vi "PID_Separate.vi"() -> ()   [LabVIEW 2018]
uses:
  <vilib>/addons/control/pid/NI_PID_pid.lvlib
  <vilib>/addons/control/pid/pid.llb/PID (DBL).vi
panel:
  in  "Reset Encoders":bool
  in  "Vasen":dbl format="%.2f"
  in  "Oikea":dbl format="%.2f"
  in  "Taka":dbl format="%.2f"
  in  "Etu":dbl format="%.2f"
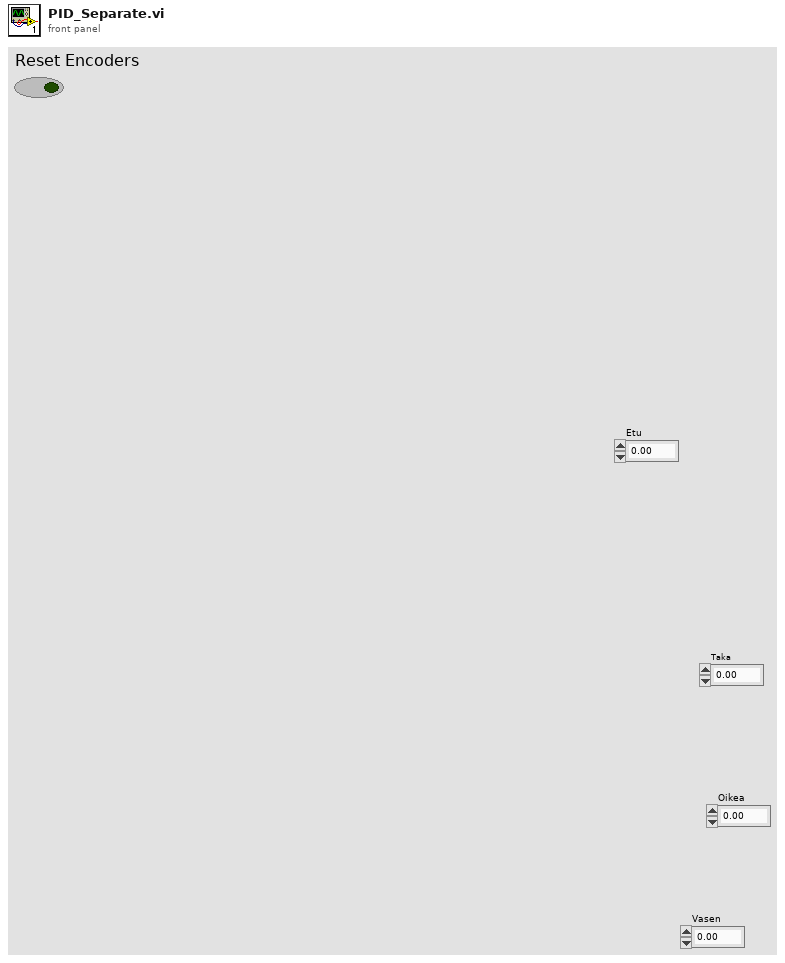
[diagram p1: front panel]
types:
  T1 = cluster{bool, "Tick Count(uSec)":u32, "Counter Value":i32[], "x-y":i32[]}
  T2 = cluster{"Position":i32[], "Velocity RPM":dbl[], "Velocity RPS":dbl[], "Radians/s":dbl[]}
  T3 = cluster{"proportional gain (Kc)":dbl, "integral time (Ti, min)":dbl, "derivative time (Td, min)":dbl}
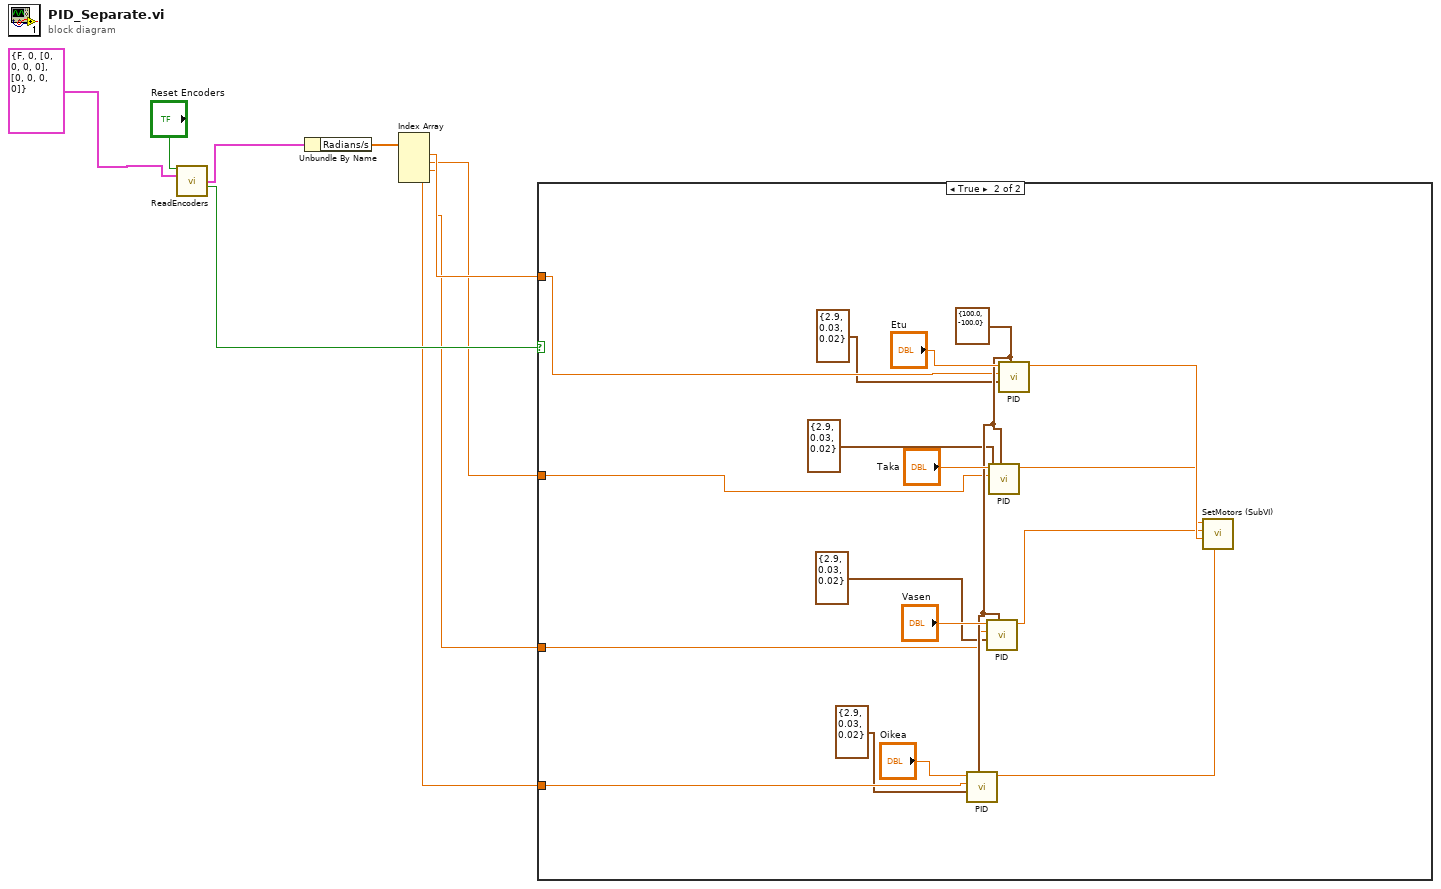
[diagram p0: block diagram]
diagram:
  n1 = call "ReadEncoders.vi"("Reset Encoders"="Reset Encoders", "Cluster in"=T1 {FALSE, "Tick Count(uSec)"=0, "Counter Value"=[0, 0, 0, 0], "x-y"=[0, 0, 0, 0]}) -> ("output cluster"=w6:T2, "Updated"=w8:bool)  [unwired: 9 in, 3 out]
  n2 = Unbundle By Name(w6) -> ("Radians/s"=w5:dbl[])
  n3 = Index Array(array=w5) -> (element #1=w4:dbl, element #2=w3:dbl, element #3=w2:dbl, element #4=w1:dbl)  [unwired: 4 in]
  n4 = case shown="True" w8 {
    tunnel: w4 -> [_ w17]
    tunnel: w3 -> [_ w16]
    tunnel: w2 -> [_ w15]
    tunnel: w1 -> [_ w14]
    frame False {
    }
    frame True {
      w18 = cluster{"output high":dbl, "output low":dbl} {"output high"=100.0, "output low"=-100.0} ("output range")
      n5 = call-poly <vilib>:"PID.vi"("output range"=w18, "PID gains"=T3 {"proportional gain (Kc)"=2.9, "integral time (Ti, min)"=0.03, "derivative time (Td, min)"=0.02}, "process variable"=w14, "setpoint"="Oikea") -> ("output"=w19:dbl)  [unwired: 6 in, 1 out]
      n6 = call-poly <vilib>:"PID.vi"("output range"=w18, "PID gains"=T3 {"proportional gain (Kc)"=2.9, "integral time (Ti, min)"=0.03, "derivative time (Td, min)"=0.02}, "process variable"=w15, "setpoint"="Vasen") -> ("output"=w20:dbl)  [unwired: 6 in, 1 out]
      n7 = call-poly <vilib>:"PID.vi"("output range"=w18, "PID gains"=T3 {"proportional gain (Kc)"=2.9, "integral time (Ti, min)"=0.03, "derivative time (Td, min)"=0.02}, "process variable"=w16, "setpoint"="Taka") -> ("output"=w21:dbl)  [unwired: 6 in, 1 out]
      n8 = call-poly <vilib>:"PID.vi"("output range"=w18, "PID gains"=T3 {"proportional gain (Kc)"=2.9, "integral time (Ti, min)"=0.03, "derivative time (Td, min)"=0.02}, "process variable"=w17, "setpoint"="Etu") -> ("output"=w22:dbl)  [unwired: 6 in, 1 out]
      n9 = call "SetMotors (SubVI).vi"("Oikea"=w19, "Etu"=w22, "Vasen"=w20, "Taka"=w21) -> ()  [unwired: 8 in]
    }
  }
